vi "V7310.File.Write.vi"(8 "error in":errorcluster, 11 "SettingsPath":path=path "D:/work/WABCO/LV-MIX/SOFTWARE/settings") -> (0 "error out":errorcluster)   [LabVIEW 2016]
uses:
  tools/Tma.lib/nlconfig.llb/fp2ini mode.ctl
  V7310.Global.vi
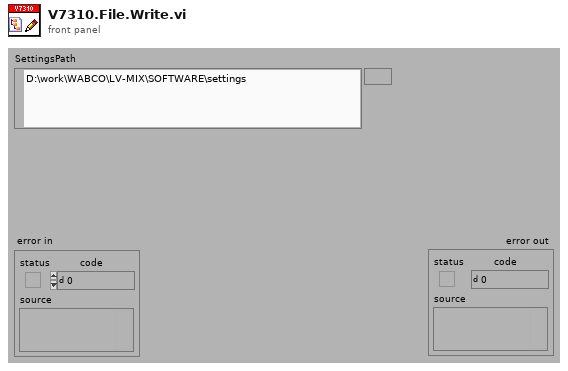
[diagram p1: front panel]
types:
  T1 = typedef "V7310.Data.Status.ctl" = cluster{"State":T2, "LaserStatus":T3, "LaserStatusRaw":string, "Ref":refnum<k5>, "RTC TS":timestamp, "Conn TS":timestamp, "Msg":T4[], "JobInUse":string, "Jobs":string[], "Vars":T5[]}
  T2 = typedef "V7310.Data.Status.State.ctl" = enum16{"First", "Init", "Msg", "Error", "Abort", "Idle", "Run"}
  T3 = typedef "V7310.LaserStatus.ctl" = enum16{"-", "FatalError", "Initialize", "KeySwitchOpen", "TimeoutInterlock", "InterlockOpen", "StartUp", "ShutterlockOpen", "Standby", "Ready", "PrepareForMarking", "WaitForTrigger", "Marking"}
  T4 = typedef "V7310.Message.Data.ctl" = cluster{"ID":i32, "Msg":string}
  T5 = typedef "V7310.Job.Variable.ctl" = cluster{"Name":string, "Value":string}
  T6 = typedef "fp2ini mode.ctl" = enum16{"Read Controls", "Write Controls", "Write Indicators", "Read Indicators", "Write all", "Read all"}
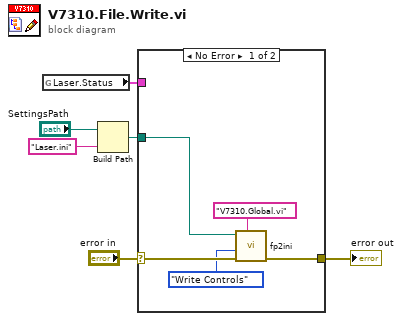
[diagram p0: block diagram]
diagram:
  n1 = global read "V7310.Global.vi" "Laser.Status"() -> (w3:T1)
  n2 = Build Path(base path="SettingsPath", name or relative path="Laser.ini") -> (appended path=w6:path)
  n3 = case shown="No Error" "error in" {
    selector: "error in" -> [w10 w12]
    tunnel: [w11 w12] -> w4
    tunnel: w6 -> [w9 _]
    tunnel: w3 -> [_ _]
    frame No Error {
      n4 = call "fp2ini.vi"("vi-name (caller if empty)"="V7310.Global.vi", "error in"=w10, "mode"=fp2ini_mode."Write Controls", "ini-file path"=w9) -> ("error out"=w11:errorcluster)  [unwired: 3 in, 4 out]
    }
    frame Error {
    }
  }
  "error out" <- w4
